vi "Material-ConfigPage-SendErrorToDialog.vi"(0 "Configuration Page in":refnum<class "Material-ConfigPage.lvclass">, 11 "error in":errorcluster) -> (4 "Configuration Page out":refnum<class "Material-ConfigPage.lvclass">, 15 "error out":errorcluster)   [LabVIEW 2013, in "Material-ConfigPage.lvclass"]
uses:
  Material-ConfigPage.lvclass
panel:
  # "Inputs"
  # "Outputs"
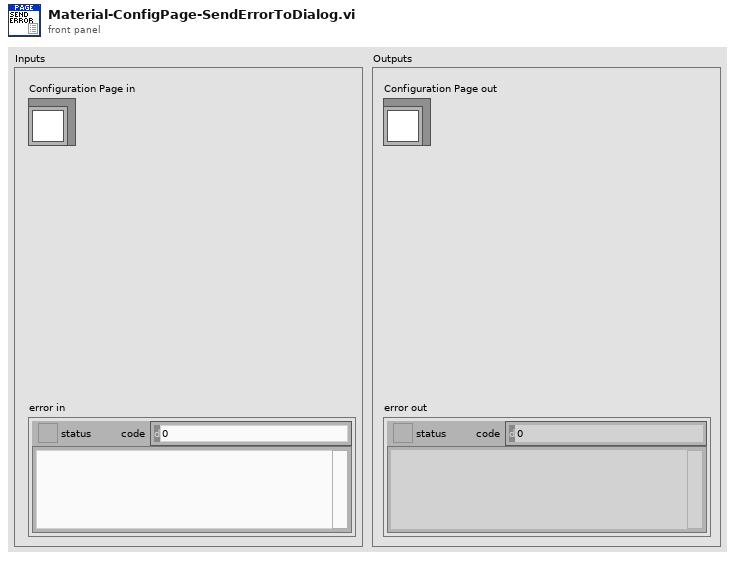
[diagram p1: front panel]
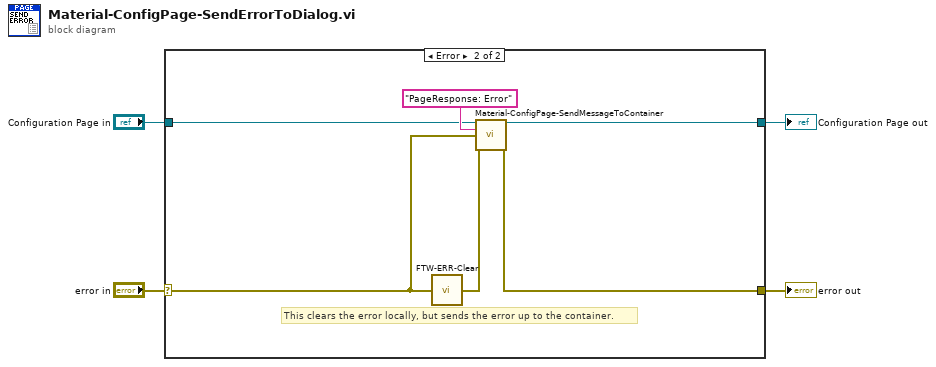
[diagram p0: block diagram]
diagram:
  n1 = case shown="Error" "error in" {
    selector: "error in" -> [w6 w8]
    tunnel: [w6 w9] -> w4
    tunnel: [w5 w10] -> w2
    tunnel: "Configuration Page in" -> [w5 w11]
    frame No Error {
    }
    frame Error {
      # "This clears the error locally, but sends the error up to the container."
      n2 = call "FTW-ERR-Clear.vi"("error to snuff"=w8) -> ("no error"=w7:errorcluster)
      n3 = call "Material-ConfigPage-SendMessageToContainer.vi"("Configuration Page"=w11, "Parameter"="PageResponse: Error", "Payload"=w8, "error in"=w7) -> ("Configuration Page out"=w10:refnum<class "Material-ConfigPage.lvclass">, "error out"=w9:errorcluster)  [unwired: 10 in]
    }
  }
  "error out" <- w4
  "Configuration Page out" <- w2
